vi "testUintDivide.vi"(8 "error in (no error)":errorcluster, 11 "TestCase in":refnum<class "UnitTestUintClass.lvclass">) -> (0 "error out":errorcluster, 3 "TestCase out":refnum<class "UnitTestUintClass.lvclass">)   [LabVIEW 2011, in "UnitTestUintClass.lvclass"]
uses:
  UnitTestUintClass.lvclass
  UnitTestUintClass.lvclass/UnitTestUintClass.ctl
  <vilib>/addons/_JKI Toolkits/VI Tester/TestCase.llb/TestCase.lvclass
  UintClass/UintClass.lvclass
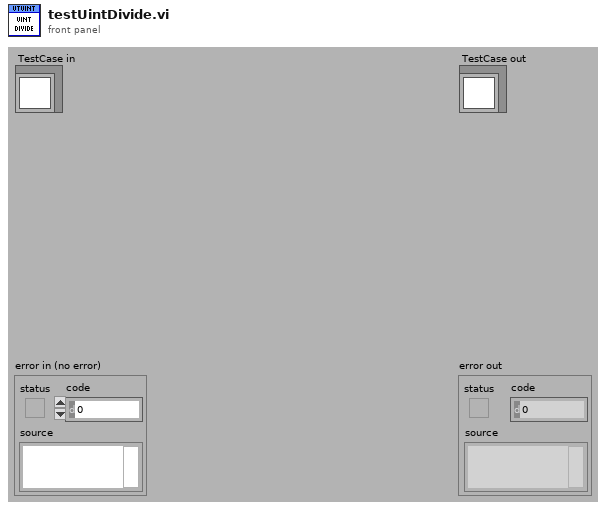
[diagram p1: front panel]
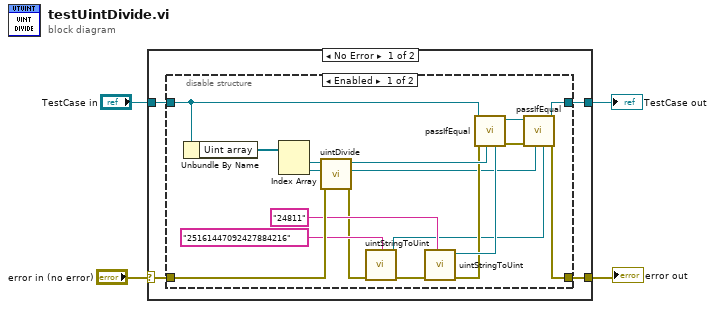
[diagram p0: block diagram]
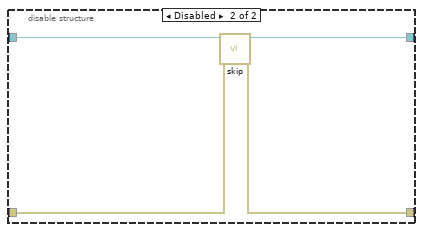
[diagram p2: hidden frame]
diagram:
  n1 = case shown="No Error" "error in (no error)" {
    selector: "error in (no error)" -> [w6 w32]
    tunnel: [w5 w32] -> w3
    tunnel: [w7 w31] -> w1
    tunnel: "TestCase in" -> [w8 w31]
    frame No Error {
      n2 = disable-structure shown="Enabled" {
        disable-tunnel: w8 -> [w26 w30]
        disable-tunnel: [w12 w27] -> w7
        disable-tunnel: w6 -> [w20 w29]
        disable-tunnel: [w9 w28] -> w5
        frame Enabled {
          n3 = Unbundle By Name(w26) -> ("Uint array"=w25:refnum<class "UintClass.lvclass">[])
          n4 = Index Array(array=w25) -> (element #1=w24:refnum<class "UintClass.lvclass">, element #2=w23:refnum<class "UintClass.lvclass">)  [unwired: 2 in]
          n5 = call "uintDivide.vi"("Error in (no error)"=w20, "Uint2 in"=w23, "Uint1 in"=w24) -> ("Error out"=w15:errorcluster, "floor(Uint1/Uint2)"=w11:refnum<class "UintClass.lvclass">, "Uint1 mod Uint2"=w22:refnum<class "UintClass.lvclass">)  [unwired: 5 in, 1 out]
          n6 = call "uintStringToUint.vi"("Error in (no error)"=w15, "String in"="25161447092427884216") -> ("Error out"=w16:errorcluster, "Uint out"=w10:refnum<class "UintClass.lvclass">)  [unwired: 8 in]
          n7 = call "uintStringToUint.vi"("Error in (no error)"=w16, "String in"="24811") -> ("Error out"=w19:errorcluster, "Uint out"=w21:refnum<class "UintClass.lvclass">)  [unwired: 8 in]
          n8 = call-dynamic "passIfEqual.vi"("error in (no error)"=w19, "y"=w21, "x"=w22, "TestCase in"=w26) -> ("error out"=w14:errorcluster, "TestCase out"=w13:refnum<class "UnitTestUintClass.lvclass">)  [unwired: 6 in]
          n9 = call-dynamic "passIfEqual.vi"("error in (no error)"=w14, "y"=w10, "x"=w11, "TestCase in"=w13) -> ("error out"=w9:errorcluster, "TestCase out"=w12:refnum<class "UnitTestUintClass.lvclass">)  [unwired: 6 in]
        }
        frame Disabled {
          n10 = call <vilib>:"skip.vi"("error in (no error)"=w29, "TestCase in"=w30) -> ("error out"=w28:errorcluster, "TestCase out"=w27:refnum<class "UnitTestUintClass.lvclass">)  [unwired: 8 in]
        }
      }
    }
    frame Error {
    }
  }
  "error out" <- w3
  "TestCase out" <- w1
